vi "PhysicsDialog.vi"() -> ()   [LabVIEW 2020]
uses:
  global/SettingVariable.vi
  <vilib>/Utility/config.llb/Write Key (Double).vi
  global/GlobalVariable.vi
  <vilib>/Utility/config.llb/NI_LVConfig.lvlib
panel:
  in  "下发":bool
  in  "Lambda 6":sgl caption="Lambda 6:"
  in  "Lambda 5":sgl caption="Lambda 5:"
  in  "Lambda 4":sgl caption="Lambda 4:"
  in  "Lambda 3":sgl caption="Lambda 3:"
  in  "Lambda 2":sgl caption="Lambda 2:"
  in  "βeff 6":sgl caption="βeff 6:"
  in  "βeff 5":sgl caption="βeff 5:"
  in  "βeff 4":sgl caption="βeff 4:"
  in  "βeff 3":sgl caption="βeff 3:"
  in  "βeff 2":sgl caption="βeff 2:"
  in  "取消":bool caption="Cancel Button"
  in  "确定":bool
  in  "Lambda 1":sgl caption="Lambda 1:"
  in  "βeff 1":sgl caption="βeff 1:"
  in  "源强":sgl caption="源强(n/cm2·s):"
  in  "中子寿命":sgl caption="中子寿命(s):"
  # "中子学参数"
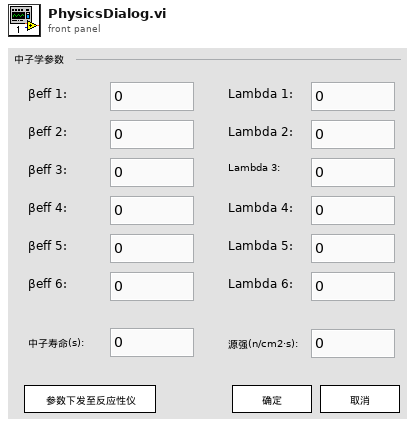
[diagram p1: front panel]
types:
  T1 = enum16{"fractional", "engineering", "exponential"}
  T2 = typedef "NI_LVConfig.lvlib/Config Data RefNum.ctl" = refnum<k1>
  T3 = enum32{"Bad", "Idle", "Run top level", "Running"}
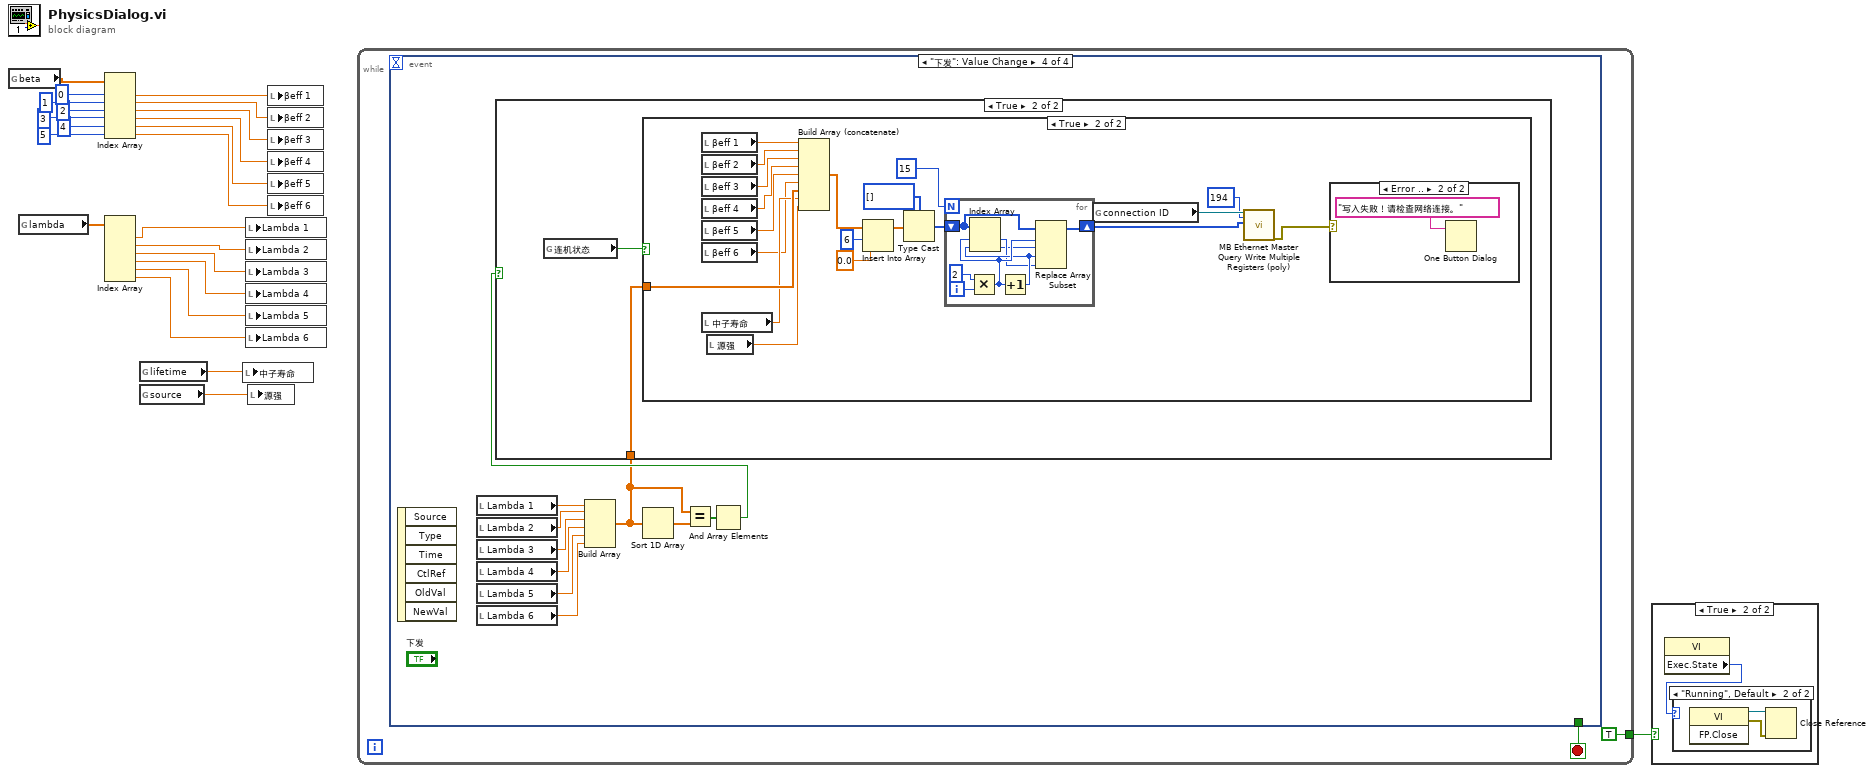
[diagram p0: block diagram]
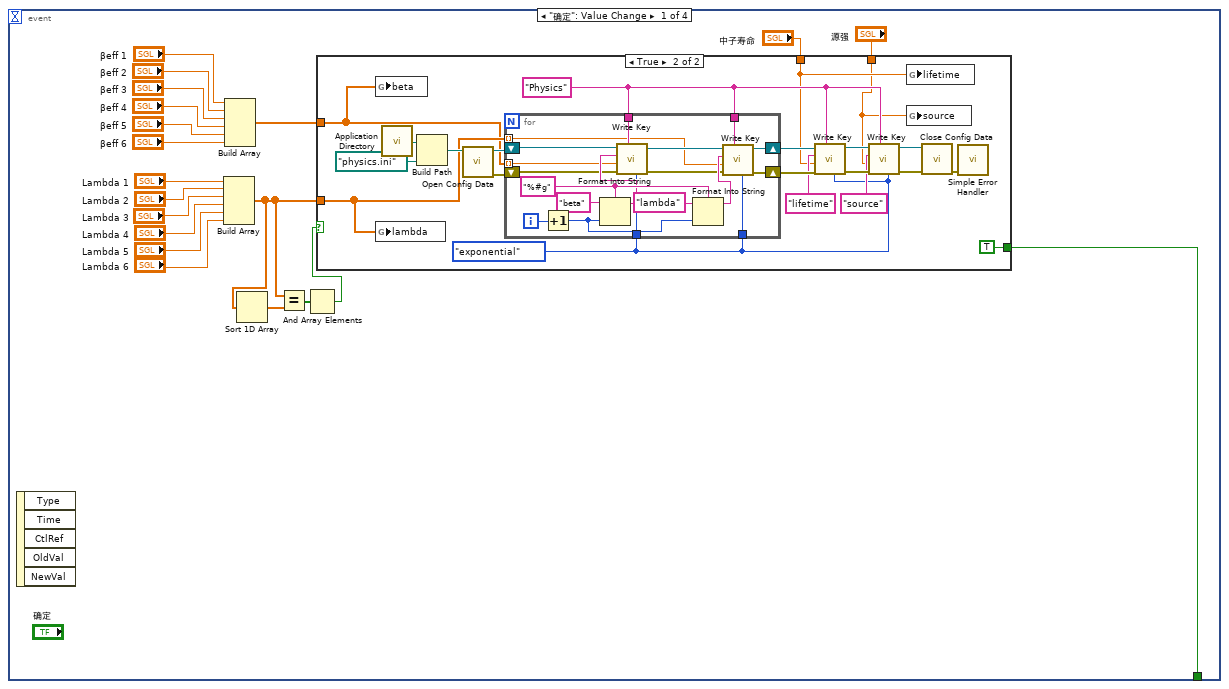
[diagram p4: hidden frame]
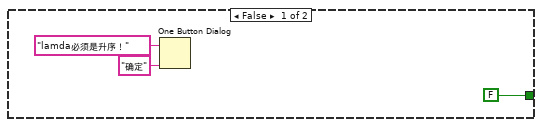
[diagram p5: hidden frame]
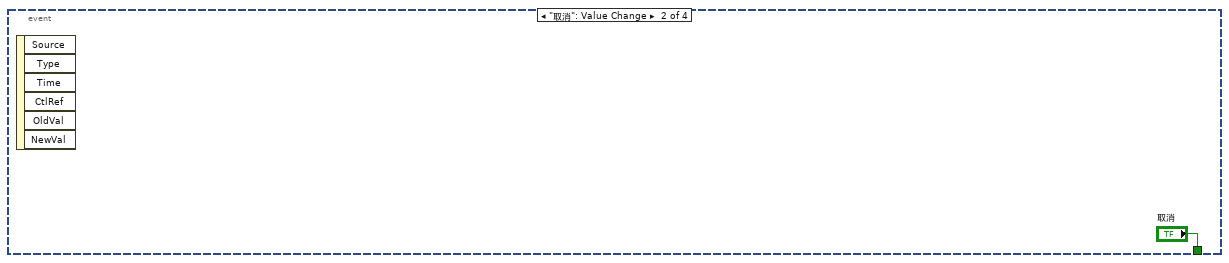
[diagram p6: hidden frame]
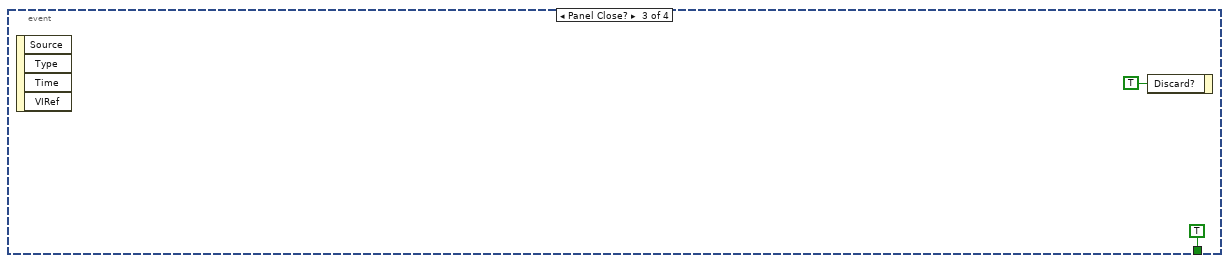
[diagram p7: hidden frame]
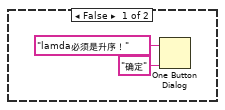
[diagram p8: hidden frame]
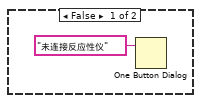
[diagram p9: hidden frame]
diagram:
  n1 = global read "SettingVariable.vi" "beta"() -> (w9:dbl[])
  n2 = global read "SettingVariable.vi" "lambda"() -> (w10:dbl[])
  n3 = Index Array(array=w9, index #1=0, index #2=1, index #3=2, index #4=3, index #5=4, index #6=5) -> (element #1=w17:dbl, element #2=w16:dbl, element #3=w15:dbl, element #4=w14:dbl, element #5=w13:dbl, element #6=w12:dbl)
  n4 = Index Array(array=w10) -> (element #1=w3:dbl, element #2=w4:dbl, element #3=w5:dbl, element #4=w6:dbl, element #5=w7:dbl, element #6=w8:dbl)  [unwired: 6 in]
  n5 = global read "SettingVariable.vi" "lifetime"() -> (w2:dbl)
  n6 = global read "SettingVariable.vi" "source"() -> (w1:dbl)
  n7 = local write "中子寿命"(w2) -> ()
  n8 = local write "Lambda 1"(w3) -> ()
  n9 = local write "Lambda 2"(w4) -> ()
  n10 = local write "Lambda 3"(w5) -> ()
  n11 = local write "Lambda 4"(w6) -> ()
  n12 = local write "Lambda 5"(w7) -> ()
  n13 = local write "Lambda 6"(w8) -> ()
  n14 = local write "源强"(w1) -> ()
  n15 = local write "βeff 1"(w17) -> ()
  n16 = local write "βeff 2"(w16) -> ()
  n17 = local write "βeff 3"(w15) -> ()
  n18 = local write "βeff 4"(w14) -> ()
  n19 = local write "βeff 5"(w13) -> ()
  n20 = local write "βeff 6"(w12) -> ()
  n21 = while {
    tunnel: [TRUE ("确定")] -> w11
    stop <- w25 stop-if-true
    n22 = event shown="[3] \"下发\": Value Change" {
      selector: _ -> [_ _ _ _]
      dyn-events: _ -> [_ _ _ _]
      timeout: _ -> [_ _ _ _]
      tunnel: [w26 "取消" TRUE ("确定") _] -> w25
      event "确定": Value Change {
        n23 = event-data() -> ()  [unwired: 1 in, 5 out]
        n24 = Build Array("Lambda 1", "Lambda 2", "Lambda 3", "Lambda 4", "Lambda 5", "Lambda 6") -> (w30:sgl[])
        n25 = Build Array("βeff 1", "βeff 2", "βeff 3", "βeff 4", "βeff 5", "βeff 6") -> (w33:sgl[])
        n26 = Sort 1D Array(array=w30) -> (sorted array=w29:sgl[])
        n27 = Equal?(x=w30, y=w29) -> (x = y?=w28:bool[])
        n28 = And Array Elements(Boolean array=w28) -> (logical AND=w27:bool)
        n29 = case shown="True" w27 {
          tunnel: w33 -> [_ w53]
          tunnel: w30 -> [_ w54]
          tunnel: "中子寿命" -> [_ w52]
          tunnel: "源强" -> [_ w51]
          tunnel: [FALSE ("确定") TRUE ("确定")] -> w26
          frame False {
            n30 = One Button Dialog(message="lamda必须是升序！", button name ("OK")="确定") -> ()  [unwired: 1 out]
          }
          frame True {
            w49 = T1."exponential" ("format (fractional)")
            w63 = "Physics" ("initial string")
            n31 = global write "SettingVariable.vi" "beta"(w53) -> ()
            n32 = global write "SettingVariable.vi" "lambda"(w54) -> ()
            n33 = call <vilib>:"Application Directory.vi"() -> ("Application Directory"=w68:path)
            n34 = Build Path(base path=w68, name or relative path=path "physics.ini") -> (appended path=w67:path)
            n35 = call <vilib>:"Open Config Data.vi"("configuration file path"=w67) -> ("error out"=w65:errorcluster, "refnum"=w66:T2)  [unwired: 2 in, 7 out]
            n36 = for {
              tunnel: w63 -> [w81]
              tunnel: w63 -> [w80]
              tunnel: w53 -> [w79] mode=indexing
              tunnel: w54 -> [w74] mode=indexing
              shift-right: [w72] -> w62
              shift-left: w66 -> [w78]
              shift-right: [w73] -> w60
              shift-left: w65 -> [w77]
              tunnel: w49 -> [w71]
              tunnel: w49 -> [w70]
              i -> [w88]
              w84 = "%#g" ("section")
              n37 = Increment(x=w88) -> (x+1=w85:i32)
              n38 = Format Into String(format string=w84, initial string="beta", w85) -> (resulting string=w83:string)  [unwired: 1 in, 1 out]
              n39 = call-poly <vilib>:"Write Key.vi"("format (fractional)"=w71, "section"=w81, "error in (no error)"=w77, "value"=w79, "key"=w83, "refnum"=w78) -> ("error out"=w76:errorcluster, "refnum out"=w75:T2)  [unwired: 3 in, 1 out]
              n40 = Format Into String(format string=w84, initial string="lambda", w85) -> (resulting string=w82:string)  [unwired: 1 in, 1 out]
              n41 = call-poly <vilib>:"Write Key.vi"("format (fractional)"=w70, "section"=w80, "error in (no error)"=w76, "value"=w74, "key"=w82, "refnum"=w75) -> ("error out"=w73:errorcluster, "refnum out"=w72:T2)  [unwired: 3 in, 1 out]
            }
            n42 = call-poly <vilib>:"Write Key.vi"("format (fractional)"=w49, "section"=w63, "error in (no error)"=w60, "value"=w52, "key"="lifetime", "refnum"=w62) -> ("error out"=w59:errorcluster, "refnum out"=w61:T2)  [unwired: 3 in, 1 out]
            n43 = call-poly <vilib>:"Write Key.vi"("format (fractional)"=w49, "section"=w63, "error in (no error)"=w59, "value"=w51, "key"="source", "refnum"=w61) -> ("error out"=w57:errorcluster, "refnum out"=w58:T2)  [unwired: 3 in, 1 out]
            n44 = global write "SettingVariable.vi" "lifetime"(w52) -> ()
            n45 = global write "SettingVariable.vi" "source"(w51) -> ()
            n46 = call <vilib>:"Close Config Data.vi"("error in (no error)"=w57, "refnum"=w58) -> ("error out"=w64:errorcluster)  [unwired: 1 in, 8 out]
            n47 = call <vilib>:"Simple Error Handler.vi"("error in (no error)"=w64) -> ()  [unwired: 1 in, 8 out]
          }
        }
      }
      event "取消": Value Change {
        n48 = event-data() -> ()  [unwired: 1 in, 6 out]
      }
      event Panel Close? {
        n49 = event-data() -> ()  [unwired: 1 in, 4 out]
        n50 = event-data("Discard?"=TRUE) -> ()  [unwired: 1 in, 1 out]
      }
      event "下发": Value Change {
        n51 = event-data() -> ()  [unwired: 1 in, 6 out]
        n52 = local read "Lambda 1"() -> (w101:sgl)
        n53 = local read "Lambda 2"() -> (w100:sgl)
        n54 = local read "Lambda 3"() -> (w99:sgl)
        n55 = local read "Lambda 4"() -> (w98:sgl)
        n56 = local read "Lambda 5"() -> (w97:sgl)
        n57 = local read "Lambda 6"() -> (w96:sgl)
        n58 = Build Array(w101, w100, w99, w98, w97, w96) -> (w92:sgl[])
        n59 = Sort 1D Array(array=w92) -> (sorted array=w95:sgl[])
        n60 = Equal?(x=w92, y=w95) -> (x = y?=w94:bool[])
        n61 = And Array Elements(Boolean array=w94) -> (logical AND=w93:bool)
        n62 = case shown="True" w93 {
          tunnel: w92 -> [_ w104]
          frame False {
            n63 = One Button Dialog(message="lamda必须是升序！", button name ("OK")="确定") -> ()  [unwired: 1 out]
          }
          frame True {
            n64 = global read "GlobalVariable.vi" "连机状态"() -> (w105:bool)
            n65 = case shown="True" w105 {
              tunnel: w104 -> [_ w124]
              frame False {
                n66 = One Button Dialog(message="未连接反应性仪") -> ()  [unwired: 1 in, 1 out]
              }
              frame True {
                n67 = local read "βeff 1"() -> (w126:sgl)
                n68 = local read "βeff 2"() -> (w125:sgl)
                n69 = local read "βeff 3"() -> (w121:sgl)
                n70 = local read "βeff 4"() -> (w120:sgl)
                n71 = local read "βeff 5"() -> (w119:sgl)
                n72 = local read "βeff 6"() -> (w118:sgl)
                n73 = local read "中子寿命"() -> (w123:sgl)
                n74 = local read "源强"() -> (w122:sgl)
                n75 = Build Array (concatenate)(w126, w125, w121, w120, w119, w118, w124, w123, w122) -> (w111:sgl[])
                n76 = Insert Into Array(array=w111, index=6 ("索引"), new element=sgl 0.0 ("新元素/子数组")) -> (w117:sgl[])
                n77 = Type Cast(type=u16[] [] ("Input Registers"), x=w117) -> (*(type *) &x=w116:u16[])
                n78 = for {
                  N: 15 -> [_]
                  shift-right: [w128] -> w109
                  shift-left: w116 -> [w133]
                  i -> [w135]
                  n79 = Multiply(x=2, y=w135) -> (x*y=w132:i32)
                  n80 = Increment(x=w132) -> (x+1=w131:i32)
                  n81 = Index Array(array=w133, index #1=w132, index #2=w131) -> (element #1=w130:u16, element #2=w129:u16)
                  n82 = Replace Array Subset(array=w133, new element #1=w129, index #1=w132, new element #2=w130, index #2=w131) -> (w128:u16[])
                }
                n83 = global read "GlobalVariable.vi" "connection ID"() -> (w110:refnum<k5>)
                n84 = call "MB Ethernet Master Query Write Multiple Registers (poly).vi"("TCP Connection Refnum in"=w110, "Starting Address"=u16 194, "Registers"=w109) -> ("error out"=w107:errorcluster)  [unwired: 14 in, 2 out]
                n85 = case shown="Error .." w107 {
                  frame No Error {
                  }
                  frame Error {
                    n86 = One Button Dialog(message="写入失败！请检查网络连接。") -> ()  [unwired: 1 in, 1 out]
                  }
                }
              }
            }
          }
        }
      }
    }
  }
  n87 = case shown="True" w11 {
    frame False {
    }
    frame True {
      n88 = property class="VI"() -> ("Exec.State"=w136:T3)  [unwired: 2 in, 2 out]
      n89 = case shown="\"Running\", Default" w136 {
        frame "Run top level" {
        }
        frame "Running", Default {
          n90 = invoke class="VI" method="FP.Close"() -> (reference out=w137:refnum<vi>, error out=w138:errorcluster)  [unwired: 3 in, 1 out]
          n91 = Close Reference(reference=w137, error in (no error)=w138) -> ()  [unwired: 1 out]
        }
      }
    }
  }
